vi "draw.picture.vi"(10 "picture data":T1, 11 "picture in":picture) -> (1 "enddate":dbl, 2 "startdate":dbl, 3 "picture":picture)   [LabVIEW 2024]
uses:
  picture.data--cluster.ctl
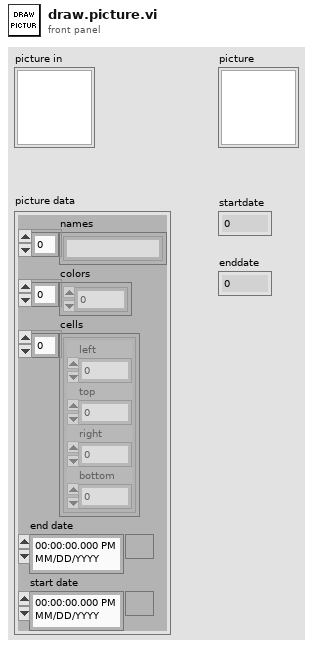
[diagram p1: front panel]
types:
  T1 = typedef "picture.data--cluster.ctl" = cluster{"names":string[], "colors":u32[], "cells":cluster{"left":i16, "top":i16, "right":i16, "bottom":i16}[], "end date":timestamp, "start date":timestamp}
  T2 = cluster{"left":i16, "top":i16, "right":i16, "bottom":i16}[]
  T3 = enum16{"None", "Stacked", "Clockwise", "Counterclockwise"}
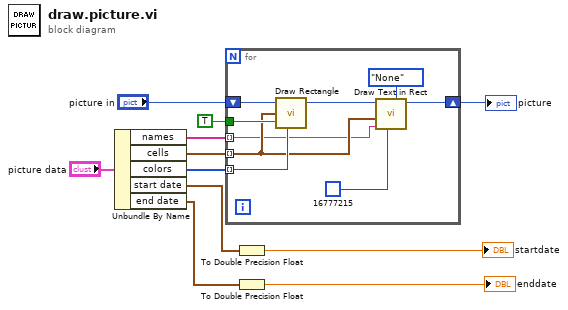
[diagram p0: block diagram]
diagram:
  n1 = Unbundle By Name("picture data") -> ("names"=w3:string[], "cells"=w5:T2, "colors"=w11:u32[], "start date"=w8:timestamp, "end date"=w9:timestamp)
  n2 = for {
    tunnel: w5 -> [w15] mode=indexing
    shift-right: [w16] -> w7
    shift-left: "picture in" -> [w20]
    tunnel: TRUE ("fill?(F)") -> [w19]
    tunnel: w11 -> [w18] mode=indexing
    tunnel: w3 -> [w14] mode=indexing
    n3 = call <vilib>:"Draw Rectangle.vi"("picture"=w20, "rect"=w15, "fill?(F)"=w19, "color(black)"=w18) -> ("new picture"=w17:picture)  [unwired: 5 in]
    n4 = call <vilib>:"Draw Text in Rect.vi"("text color(black)"=u32 16777215, "text"=w14, "rect"=w15, "text orientation"=T3."None", "picture"=w17) -> ("new picture"=w16:picture)  [unwired: 6 in]
  }
  "picture" <- w7
  n5 = To Double Precision Float(number=w8) -> (double precision float=→"startdate":dbl)
  n6 = To Double Precision Float(number=w9) -> (double precision float=→"enddate":dbl)
